vi "TurretVariable.vi"() -> ()   [LabVIEW 2020]
panel:
  out "AutoHood":dbl
  out "EncoderHoodSetpoint":dbl
  out "AutoAiming":bool
  out "EncoderTurretSetpoint":dbl
  out "Enable Aiming":bool
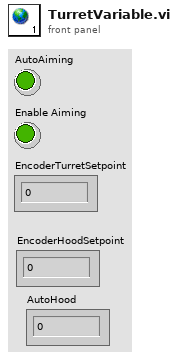
[diagram p1: front panel]
diagram:
